vi "Convert LabVIEW Colour To SDL Colour.vi"(11 "Color":u32(colorbox)) -> (3 "SDL Colour":u32 format="%.0x")   [LabVIEW 2014, in "LibSDL2.lvlib"]
uses:
  LibSDL2.lvlib
panel:
  # "LabVIEW: RGB0\nSDL: 0BGR"
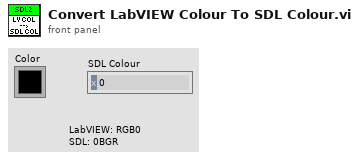
[diagram p1: front panel]
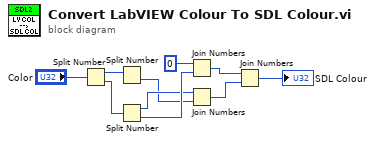
[diagram p0: block diagram]
diagram:
  n1 = Split Number(x="Color") -> (hi(x)=w1:u16, lo(x)=w2:u16)
  n2 = Split Number(x=w1) -> (lo(x)=w7:u8)  [unwired: 1 out]
  n3 = Split Number(x=w2) -> (hi(x)=w9:u8, lo(x)=w10:u8)
  n4 = Join Numbers(hi=u8 0, lo=w10) -> ((hi.lo)=w3:u16)
  n5 = Join Numbers(hi=w9, lo=w7) -> ((hi.lo)=w4:u16)
  n6 = Join Numbers(hi=w3, lo=w4) -> ((hi.lo)=→"SDL Colour":u32)
